vi "Get Required Buffer Size.vi"(8 "error in (no error)":errorcluster, 11 "Transfer Group in":refnum<class "Transfer Group.lvclass">) -> (0 "error out":errorcluster, 2 "required buffer size":u64 format="%d bytes", 3 "Transfer Group out":refnum<class "Transfer Group.lvclass">)   [LabVIEW 2017, in "Data Sharing Framework Core.lvlib" / "Data Sharing Framework Engine.lvlib" / "Transfer Group.lvclass"]
uses:
  Transfer Group.lvclass
  Transfer Group.lvclass/Transfer Group.ctl
  Transfer/Transfer.lvclass
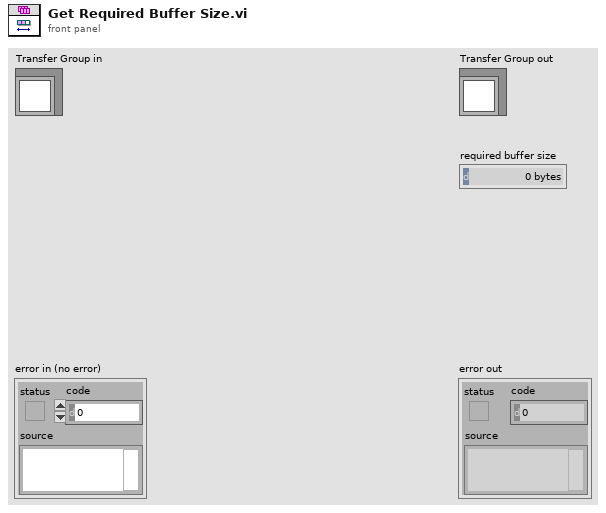
[diagram p1: front panel]
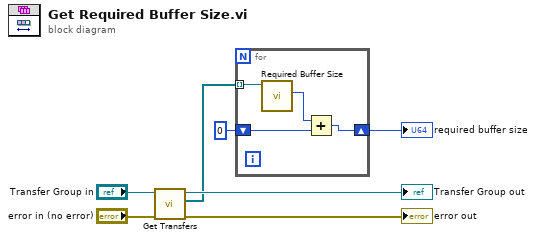
[diagram p0: block diagram]
diagram:
  n1 = call "Get Transfers.vi"("Transfer Group in"="Transfer Group in") -> ("Transfers"=w1:refnum<class "Transfer.lvclass">[], "Transfer Group out"=→"Transfer Group out":refnum<class "Transfer Group.lvclass">)  [unwired: 9 in]
  n2 = for {
    tunnel: w1 -> [w10] mode=indexing
    shift-right: [w8] -> w2
    shift-left: u64 0 -> [w7]
    n3 = call "Required Buffer Size.vi"("Transfer in"=w10) -> ("required buffer size"=w9:u64)  [unwired: 8 in, 2 out]
    n4 = Add(x=w9, y=w7) -> (x+y=w8:u64)
  }
  "required buffer size" <- w2
  "error out" <- "error in (no error)"
